vi "Destroy.vi"(8 "error in (no error)":errorcluster, 11 "Plugin Interface in":refnum<class "Plugin Interface.lvclass">) -> (0 "error out":errorcluster)   [LabVIEW 2020, in "DSF Core.lvlib" / "Plugin Interface.lvclass"]
uses:
  Plugin Interface.lvclass
  C:/Users/nitest/Desktop/Git/niveristand-data-sharing-framework-custom-device/Source/Core/Classes/Interface/Interface.lvclass
  Interface.lvclass/Interface.ctl
  Delete RT FIFO.vi
  Interface.lvclass
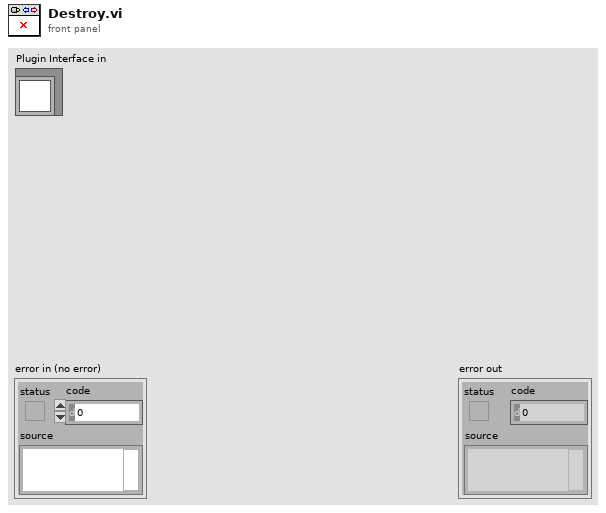
[diagram p1: front panel]
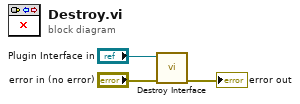
[diagram p0: block diagram]
diagram:
  n1 = call "Destroy Interface.vi"("error in (no error)"="error in (no error)", "Interface in"="Plugin Interface in") -> ("error out"=→"error out":errorcluster)  [unwired: 8 in, 1 out]
